vi "Handle Command.vi"(8 "error in (no error)":errorcluster, 9 "Data":variant, 10 "Command":string, 11 "Inst.Krohn-Hite-7008 in":refnum<class "Inst.Krohn-Hite-7008.lvclass">) -> (0 "error out":errorcluster, 1 "Processed Data":variant, 2 "Command":string, 3 "Inst.Krohn-Hite-7008 out":refnum<class "Inst.Krohn-Hite-7008.lvclass">)   [LabVIEW 2019, in "Inst.Krohn-Hite-7008.lvclass"]
uses:
  Inst.Krohn-Hite-7008.lvclass
  Typedefs/Inst.Krohn-Hite-7008.device--Cluster.ctl
  Inst.Krohn-Hite-7008.lvclass/Inst.Krohn-Hite-7008.ctl
  Typedefs/Inst.Krohn-Hite-7008.ProtectedCommands--Enum.ctl
  Typedefs/getAllChannelsResponse--Cluster.ctl
  KH7008/typedefs/allChannelProperties--Array.ctl
  KH7008/typedefs/channelProperties--Cluster.ctl
  KH7008/typedefs/channel--numeric.ctl
  KH7008/typedefs/gain--enum.ctl
  KH7008/typedefs/Input--Enum.ctl
  KH7008/typedefs/shunt--enum.ctl
  KH7008/typedefs/couple--Enum.ctl
  KH7008/typedefs/Filter--Enum.ctl
  Typedefs/Inst.Krohn-Hite-7008.Commands--Enum.ctl
  Typedefs/getChannelRequest--Cluster.ctl
  17ba76e8-dba6-4673-9f9f-19756a1b5b13.vi
  17ba76e8-dba6-4673-9f9f-19756a1b5b13.vi/2c9afdd1-6867-4b0b-b376-2fab39319be8.vi
  17ba76e8-dba6-4673-9f9f-19756a1b5b13.vi/f6a4d3ba-6616-4252-adda-9ecae78dfb9b.vi
  <vilib>/Utility/Data Type/Get Type Information.vi
  <vilib>/JDP Science/JSONtext/JSON text to Variant.vi
  <vilib>/JDP Science/JSONtext/LVClass Serializer/JSONtext LVClass Serializer.lvclass
  <userlib>/LevyLab/Instrument Framework/Instrument Types/Amplifier/Instrument.Amplifier.lvclass
  KH7008/KH7008.lvlib
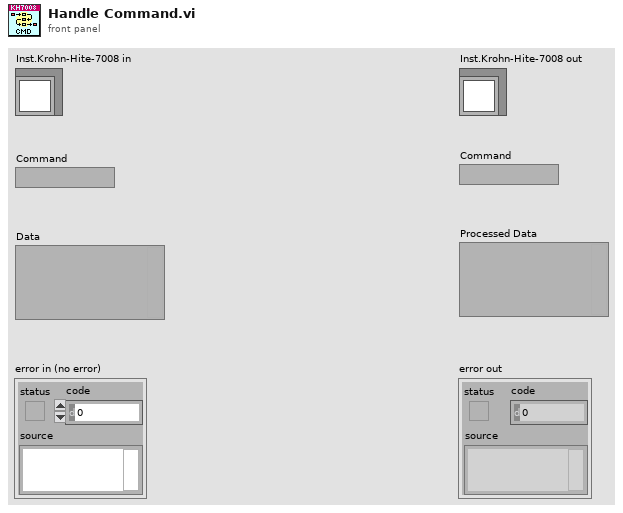
[diagram p1: front panel]
types:
  T1 = typedef "Inst.Krohn-Hite-7008.lvclass/Inst.Krohn-Hite-7008.device--Cluster.ctl" = cluster{"model":string, "device_id":string}
  T2 = typedef "Inst.Krohn-Hite-7008.lvclass/getAllChannelsResponse--Cluster.ctl" = cluster{"allChannelProperties":T3}
  T3 = typedef "KH7008.lvlib/allChannelProperties--Array.ctl" = T4[]
  T4 = typedef "KH7008.lvlib/channelProperties--Cluster.ctl" = cluster{"channel":T5, "gain":T6, "input":T7, "shunt":T8, "couple":T9, "filter":T10}
  T5 = typedef "KH7008.lvlib/channel--numeric.ctl" = u16
  T6 = typedef "KH7008.lvlib/gain--enum.ctl" = enum16{"1x", "10x", "100x", "1000x"}
  T7 = typedef "KH7008.lvlib/input--enum.ctl" = enum16{"OFF", "SE+", "SE-", "DIFF"}
  T8 = typedef "KH7008.lvlib/shunt--enum.ctl" = enum16{"Open", "50", "500", "5k", "50k", "10M"}
  T9 = typedef "KH7008.lvlib/couple--enum.ctl" = enum16{"AC", "DC"}
  T10 = typedef "KH7008.lvlib/filter--enum.ctl" = enum16{"OFF", "ON"}
  T11 = typedef "Inst.Krohn-Hite-7008.lvclass/getChannelRequest--Cluster.ctl" = cluster{"channel":T5}
  T12 = typedef "Inst.Krohn-Hite-7008.lvclass/Inst.Krohn-Hite-7008.ProtectedCommands--Enum.ctl" = enum16{"Update allChannelProperties", "Update device", "Set SR"}
  T13 = typedef "Inst.Krohn-Hite-7008.lvclass/Inst.Krohn-Hite-7008.getAll--Cluster.ctl" = cluster{"device_id":string, "model":string, "allChannelProperties_json":string, "allChannelProperties":T3}
  T14 = typedef "Inst.Krohn-Hite-7008.lvclass/Inst.Krohn-Hite-7008.Commands--Enum.ctl" = enum16{"getChannel", "getAllChannels", "setChannel", "setAllChannels"}
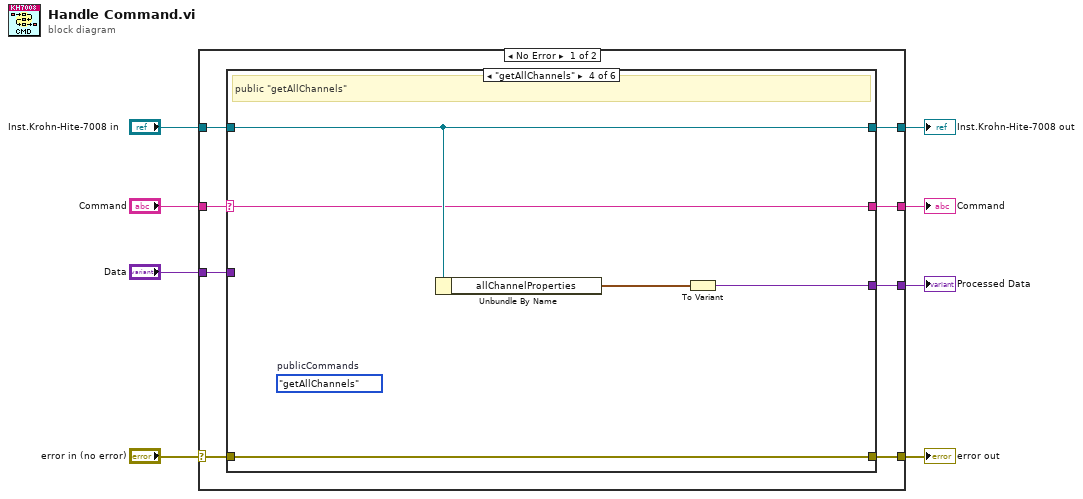
[diagram p0: block diagram]
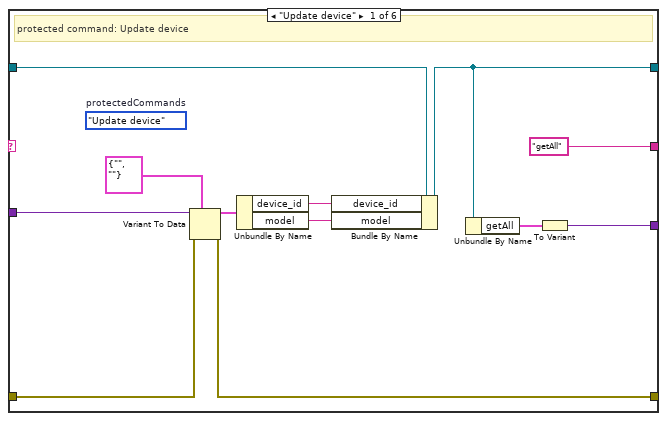
[diagram p2: hidden frame]
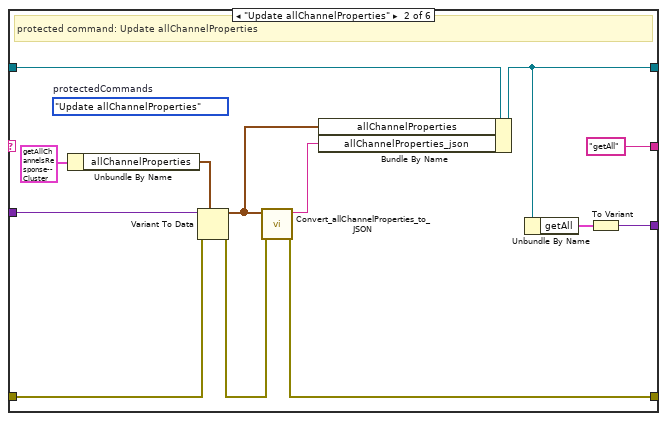
[diagram p3: hidden frame]
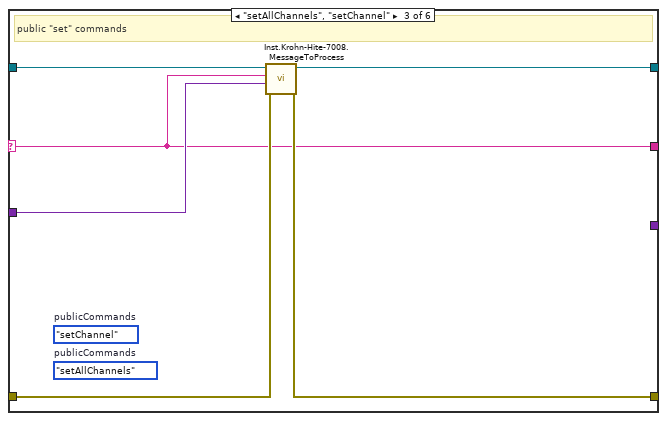
[diagram p4: hidden frame]
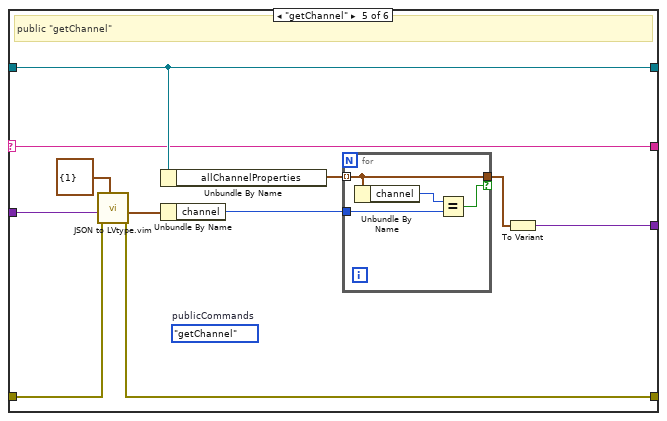
[diagram p5: hidden frame]
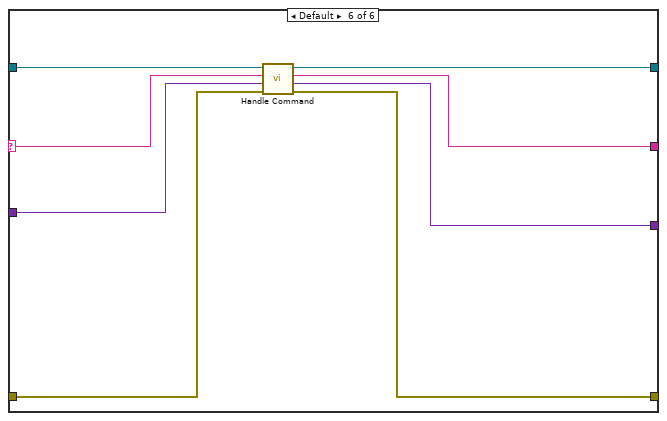
[diagram p6: hidden frame]
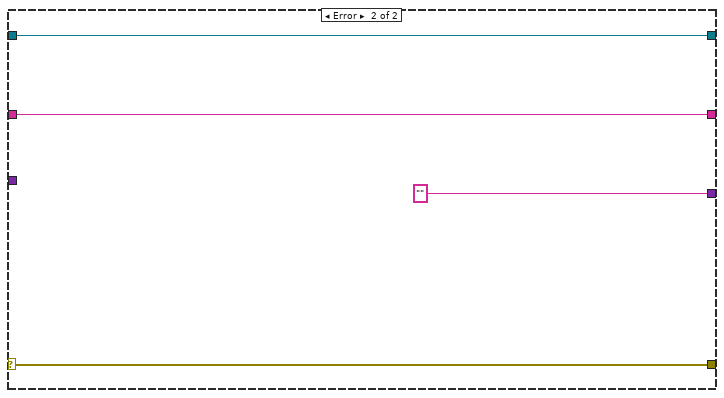
[diagram p7: hidden frame]
diagram:
  n1 = case shown="No Error" "error in (no error)" {
    selector: "error in (no error)" -> [w11 w79]
    tunnel: [w9 w79] -> w6
    tunnel: [w14 w78] -> w5
    tunnel: "Inst.Krohn-Hite-7008 in" -> [w15 w78]
    tunnel: "Command" -> [w16 w76]
    tunnel: [w13 "" ("String")] -> w3
    tunnel: "Data" -> [w10 _]
    tunnel: [w12 w76] -> w1
    frame No Error {
      n2 = case shown="\"getAllChannels\"" w16 {
        selector: w16 -> [_ _ w42 w50 w53 w69]
        tunnel: w15 -> [w28 w41 w47 w52 w63 w73]
        tunnel: [w19 w30 w46 w52 w63 w70] -> w14
        tunnel: [w17 w29 _ w51 w59 w72] -> w13
        tunnel: w11 -> [w26 w39 w45 w48 w60 w74]
        tunnel: w10 -> [w27 w40 w43 _ w61 w75]
        tunnel: ["getAll" ("Command") "getAll" ("Command") w42 w50 w53 w68] -> w12
        tunnel: [w25 w33 w44 w48 w54 w71] -> w9
        frame "Update device" {
          (unwired) Inst.Krohn-Hite-7008.ProtectedCommands--Enum."Update device"  # protectedCommands
          # "protected command: Update device"
          n3 = Variant To Data(error in=w26, type=T1 {"model"="", "device_id"=""} ("Device"), Variant=w27) -> (data=w23:T1, error out=w25:errorcluster)
          n4 = Unbundle By Name(w23) -> ("device_id"=w21:string, "model"=w22:string)
          n5 = Bundle By Name(cluster=w28, "device_id"=w21, "model"=w22) -> (w19:refnum<class "Inst.Krohn-Hite-7008.lvclass">)
          n6 = Unbundle By Name(w19) -> ("getAll"=w18:T13)
          n7 = To Variant(anything=w18) -> (Variant=w17:variant)
        }
        frame "Update allChannelProperties" {
          (unwired) Inst.Krohn-Hite-7008.ProtectedCommands--Enum."Update allChannelProperties"  # protectedCommands
          # "protected command: Update allChannelProperties"
          n8 = Unbundle By Name(T2 {"allChannelProperties"=[{"channel"=1, "gain"=enum."10x", "input"=enum."OFF", "shunt"=enum."10M", "couple"=enum."AC", "filter"=enum."OFF"}, {"channel"=2, "gain"=enum."10x", "input"=enum."OFF", "shunt"=enum."10M", "couple"=enum."AC", "filter"=enum."OFF"}, {"channel"=3, "gain"=enum."10x", "input"=enum."OFF", "shunt"=enum."10M", "couple"=enum."AC", "filter"=enum."OFF"}, {"channel"=4, "gain"=enum."10x", "input"=enum."OFF", "shunt"=enum."10M", "couple"=enum."AC", "filter"=enum."OFF"}, {"channel"=5, "gain"=enum."10x", "input"=enum."OFF", "shunt"=enum."10M", "couple"=enum."AC", "filter"=enum."OFF"}, {"channel"=6, "gain"=enum."10x", "input"=enum."OFF", "shunt"=enum."10M", "couple"=enum."AC", "filter"=enum."OFF"}, {"channel"=7, "gain"=enum."10x", "input"=enum."OFF", "shunt"=enum."10M", "couple"=enum."AC", "filter"=enum."OFF"}, {"channel"=7, "gain"=enum."10x", "input"=enum."OFF", "shunt"=enum."10M", "couple"=enum."AC", "filter"=enum."OFF"}]} ("getAllChannelsResponse")) -> ("allChannelProperties"=w37:T3)
          n9 = Variant To Data(error in=w39, type=w37, Variant=w40) -> (data=w36:T3, error out=w34:errorcluster)
          n10 = call "Convert_allChannelProperties_to_JSON.vi"("error in (no error)"=w34, "allChannelProperties"=w36) -> ("error out"=w33:errorcluster, "<JSON>"=w35:string)  [unwired: 8 in]
          n11 = Bundle By Name(cluster=w41, "allChannelProperties"=w36, "allChannelProperties_json"=w35) -> (w30:refnum<class "Inst.Krohn-Hite-7008.lvclass">)
          n12 = Unbundle By Name(w30) -> ("getAll"=w31:T13)
          n13 = To Variant(anything=w31) -> (Variant=w29:variant)
        }
        frame "setAllChannels", "setChannel" {
          (unwired) Inst.Krohn-Hite-7008.Commands--Enum."setAllChannels"  # publicCommands
          (unwired) Inst.Krohn-Hite-7008.Commands--Enum."setChannel"  # publicCommands
          # "public \"set\" commands"
          n14 = call "Inst.Krohn-Hite-7008.MessageToProcess.vi"("error in (no error)"=w45, "Data"=w43, "Command"=w42, "Inst.Krohn-Hite-7008 in"=w47) -> ("error out"=w44:errorcluster, "Inst.Krohn-Hite-7008 out"=w46:refnum<class "Inst.Krohn-Hite-7008.lvclass">)  [unwired: 6 in]
        }
        frame "getAllChannels" {
          (unwired) Inst.Krohn-Hite-7008.Commands--Enum."getAllChannels"  # publicCommands
          # "public \"getAllChannels\""
          n15 = Unbundle By Name(w52) -> ("allChannelProperties"=w49:T3)
          n16 = To Variant(anything=w49) -> (Variant=w51:variant)
        }
        frame "getChannel" {
          (unwired) Inst.Krohn-Hite-7008.Commands--Enum."getChannel"  # publicCommands
          # "public \"getChannel\""
          n17 = call "JSON to LVtype.vim"("type"=T11 {"channel"=1} ("getChannelRequest"), "error in (no error)"=w60, "JSON Data in"=w61) -> ("error out"=w54:errorcluster, "Data out"=w57:T11)  [unwired: 7 in]
          n18 = Unbundle By Name(w63) -> ("allChannelProperties"=w55:T3)
          n19 = Unbundle By Name(w57) -> ("channel"=w58:T5)
          n20 = for {
            tunnel: w55 -> [w66] mode=indexing
            tunnel: w58 -> [w67]
            tunnel: [w66] -> w56 if=w65
            n21 = Unbundle By Name(w66) -> ("channel"=w64:T5)
            n22 = Equal?(x=w64, y=w67) -> (x = y?=w65:bool)
          }
          n23 = To Variant(anything=w56) -> (Variant=w59:variant)
        }
        frame Default {
          n24 = call-parent "Handle Command.vi"("error in (no error)"=w74, "params in"=w75, "command"=w69, "Instrument in"=w73) -> ("error out"=w71:errorcluster, "processed data"=w72:variant, "command out"=w68:string, "Instrument out"=w70:refnum<class "Inst.Krohn-Hite-7008.lvclass">)  [unwired: 4 in]
        }
      }
    }
    frame Error {
    }
  }
  "error out" <- w6
  "Inst.Krohn-Hite-7008 out" <- w5
  "Command" <- w1
  "Processed Data" <- w3
